vi "Initialize with Switch Parameters Core.vi"(8 "error in (no error)":errorcluster, 10 "Switch Parameters in":refnum<class "Abstract Switch Init Parameters.lvclass">, 11 "Consumer in":refnum<class "Mock %DEVICE% Consumer.lvclass">) -> (0 "error out":errorcluster, 3 "Consumer out":refnum<class "Mock %DEVICE% Consumer.lvclass">)   [LabVIEW 2017, in "Mock %DEVICE% Consumer.lvclass"]
uses:
  Mock %DEVICE% Consumer.lvclass
  Includes/CDMessaging.lvlibp/Switch/Abstract Switch Init Parameters/Abstract Switch Init Parameters.lvclass
  Mock %DEVICE% Consumer.lvclass/Mock %DEVICE% Consumer.ctl
  Consumer/Consumer.lvclass
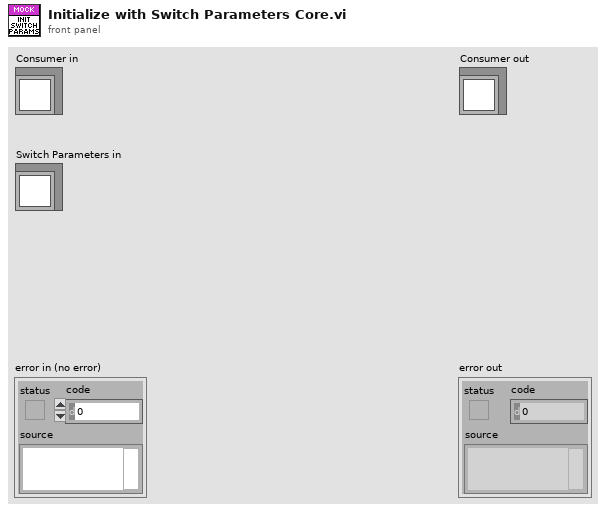
[diagram p1: front panel]
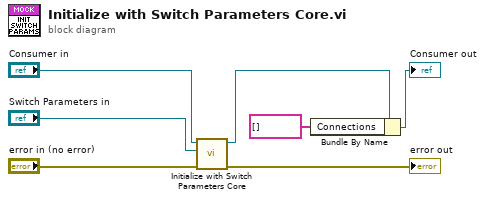
[diagram p0: block diagram]
diagram:
  n1 = call-parent "Initialize with Switch Parameters Core.vi"("error in (no error)"="error in (no error)", "Switch Parameters in"="Switch Parameters in", "Consumer in"="Consumer in") -> ("error out"=→"error out":errorcluster, "Consumer out"=w3:refnum<class "Mock %DEVICE% Consumer.lvclass">)  [unwired: 7 in]
  n2 = Bundle By Name(cluster=w3, "Connections"=string[] []) -> (→"Consumer out":refnum<class "Mock %DEVICE% Consumer.lvclass">)
